vi "Redefine Master.vi"(8 "error in (no error)":errorcluster, 11 "Master CR in":refnum<class "WebSocket Client CR.lvclass">) -> (0 "error out":errorcluster, 3 "Master CR out":refnum<class "WebSocket Client CR.lvclass">)   [LabVIEW 2021, in "WebSockets.lvlib" / "WebSocket Client CR.lvclass"]
uses:
  WebSocket Client CR.lvclass
  WebSocket Client CR.lvclass/WebSocket Client CR.ctl
  Master CR/Param/TCP Param/TCP Param.lvclass
  Master CR/Param/TCP Param/TCP Param.lvclass/TCP Param.ctl
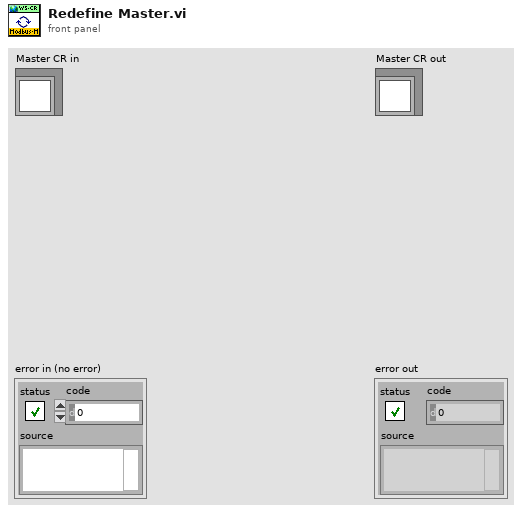
[diagram p1: front panel]
types:
  T1 = typedef "Param.lvlib/TCP Param.lvclass/timeouts.ctl" = cluster{"conn_timeout":i32, "reconn_timeout":i32, "N attempt max":i32, "t_reset_TTL":i32, "write_timeout":i32, "read_timeout":i32, "period":i32}
  T2 = cluster{"Remote IP Address":string, "Remote Port":u16}
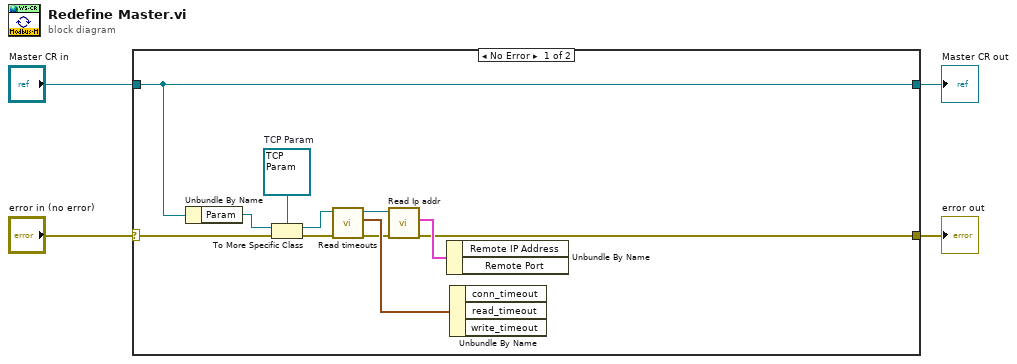
[diagram p0: block diagram]
diagram:
  n1 = case shown="No Error" "error in (no error)" {
    selector: "error in (no error)" -> [w8 w16]
    tunnel: [w5 w16] -> w1
    tunnel: [w6 w17] -> w2
    tunnel: "Master CR in" -> [w6 w17]
    frame No Error {
      w15 = refnum<class "TCP Param.lvclass"> refnum  # TCP Param
      n2 = Unbundle By Name(w6) -> ("Param"=w14:refnum<class "Param.lvclass">)
      n3 = To More Specific Class(target class=w15, reference=w14, error in=w8) -> (specific class reference=w10:refnum<class "TCP Param.lvclass">, error out=w9:errorcluster)
      n4 = call "Read timeouts.vi"("error in (no error)"=w9, "MBParam in"=w10) -> ("error out"=w7:errorcluster, "timeouts"=w11:T1, "MBParam out"=w12:refnum<class "TCP Param.lvclass">)  [unwired: 7 in]
      n5 = call "Read Ip addr.vi"("error in (no error)"=w7, "MBParam in"=w12) -> ("error out"=w5:errorcluster, "IP address"=w13:T2)  [unwired: 7 in, 1 out]
      n6 = Unbundle By Name(w13) -> ()  [unwired: 2 out]
      n7 = Unbundle By Name(w11) -> ()  [unwired: 3 out]
    }
    frame Error {
    }
  }
  "error out" <- w1
  "Master CR out" <- w2
